vi "命令解析.vi"(8 "error in (no error)":errorcluster caption="错误输入（无错误）", 10 "任务列表解析":cluster{"启用":bool, "任务":T1[]}, 11 "Cleaningcycle 输入":refnum<class "Cleaning cycle.lvclass">) -> (0 "error out":errorcluster caption="错误输出", 3 "Cleaningcycle 输出":refnum<class "Cleaning cycle.lvclass">)   [LabVIEW 2022 SP3, in "Cleaning cycle.lvclass"]
uses:
  Cleaning cycle.lvclass
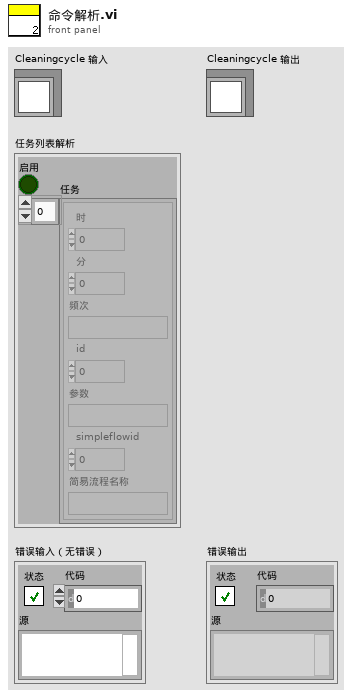
[diagram p1: front panel]
types:
  T1 = typedef "Cleaning cycle.lvclass/周期项.ctl" = cluster{"时":i32, "分":i32, "频次":string, "id":i32, "参数":string, "simpleflowid":i32, "简易流程名称":string}
  T2 = typedef "LVDateTimeRec.ctl" = cluster{"秒数的小数部分":dbl, "秒":i32, "分":i32, "时":i32, "日":i32, "月":i32, "年":i32, "天数（周）":i32, "天数（年）":i32, "DST":i32}
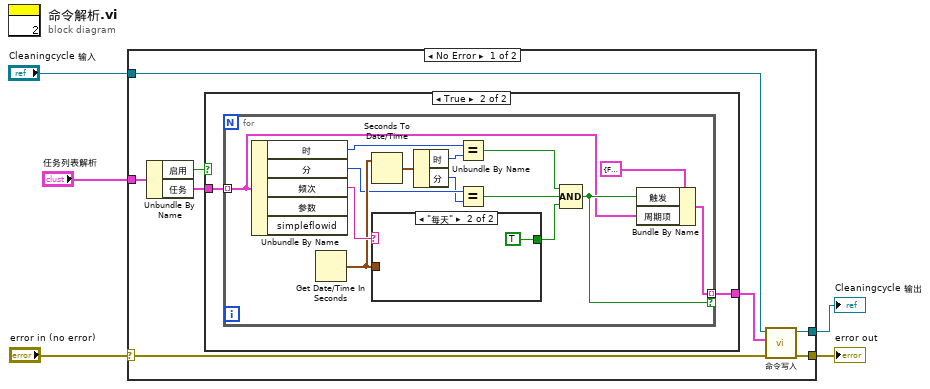
[diagram p0: block diagram]
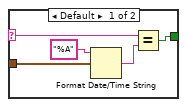
[diagram p3: hidden frame]
diagram:
  n1 = case shown="No Error" "error in (no error)" {
    selector: "error in (no error)" -> [w7 w37]
    tunnel: [w6 w37] -> w4
    tunnel: [w9 w36] -> w2
    tunnel: "Cleaningcycle 输入" -> [w10 w36]
    tunnel: "任务列表解析" -> [w13 _]
    frame No Error {
      n2 = Unbundle By Name(w13) -> ("启用"=w12:bool, "任务"=w11:T1[])
      n3 = case shown="True" w12 {
        tunnel: w11 -> [_ w15]
        tunnel: [_ w14] -> w8
        frame False {
        }
        frame True {
          n4 = for {
            tunnel: w15 -> [w16] mode=indexing
            tunnel: [w19] -> w14 mode=indexing if=w18
            n5 = Unbundle By Name(w16) -> ("时"=w24:i32, "分"=w26:i32, "频次"=w29:string)  [unwired: 2 out]
            n6 = Get Date/Time In Seconds() -> (seconds since 1Jan1904=w28:timestamp)
            n7 = Seconds To Date/Time(time stamp (now)=w28) -> (date time rec=w27:T2)  [unwired: 1 in]
            n8 = case shown="\"每天\"" w29 {
              selector: w29 -> [w31 _]
              tunnel: w28 -> [w34 _]
              tunnel: [w30 TRUE] -> w20
              frame Default {
                n9 = Format Date/Time String(time format string (%c)="%A" ("时间格式字符串(%c)"), seconds (now)=w34) -> (date/time string=w32:string)  [unwired: 1 in]
                n10 = Equal?(x=w31, y=w32) -> (x = y?=w30:bool)
              }
              frame "每天" {
              }
            }
            n11 = Unbundle By Name(w27) -> ("时"=w23:i32, "分"=w25:i32)
            n12 = Equal?(x=w24, y=w23) -> (x = y?=w22:bool)
            n13 = Equal?(x=w26, y=w25) -> (x = y?=w21:bool)
            n14 = Compound Arithmetic op=AND ("复合运算")(w22, w21, w20) -> (w18:bool)
            n15 = Bundle By Name(cluster=cluster{"触发":bool, "周期项":T1} {"触发"=FALSE, "周期项"={"时"=0, "分"=0, "频次"="", "id"=0, "参数"="", "simpleflowid"=0, "简易流程名称"=""}} ("命令"), "触发"=w18, "周期项"=w16) -> (w19:cluster{"触发":bool, "周期项":T1})
          }
        }
      }
      n16 = call "命令写入.vi"("error in (no error)"=w7, "命令"=w8, "Cleaningcycle 输入"=w10) -> ("error out"=w6:errorcluster, "Cleaningcycle 输出"=w9:refnum<class "Cleaning cycle.lvclass">)  [unwired: 7 in]
    }
    frame Error {
    }
  }
  "error out" <- w4
  "Cleaningcycle 输出" <- w2
